vi "Throw Invalid RDMA Configuration Error.vi"(7 "source vi name":string, 8 "error in":errorcluster) -> (0 "error out":errorcluster)   [LabVIEW 2020, in "RDMA.lvlib" / "RDMA Transceiver.lvclass"]
uses:
  RDMA Transceiver.lvclass
  Errors.ctl
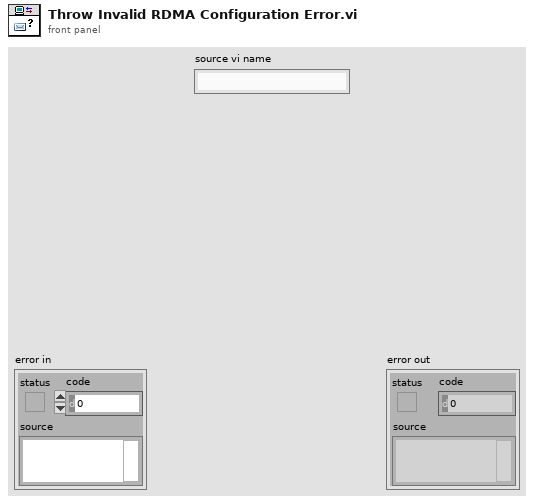
[diagram p1: front panel]
types:
  T1 = typedef "RDMA.lvlib/RDMA Transceiver.lvclass/Errors.ctl" = enum16{"Invalid RDMA Configuration", "Too Many Transfers", "Size Mismatch", "Unknown Setting"}
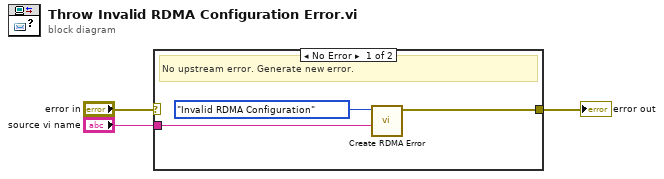
[diagram p0: block diagram]
diagram:
  n1 = case shown="No Error" "error in" {
    selector: "error in" -> [_ w7]
    tunnel: [w5 w7] -> w2
    tunnel: "source vi name" -> [w4 _]
    frame No Error {
      # "No upstream error. Generate new error."
      n2 = call "Create RDMA Error.vi"("source vi name"=w4, "error"=Errors."Invalid RDMA Configuration" ("Error")) -> ("error out"=w5:errorcluster)  [unwired: 8 in, 1 out]
    }
    frame Error {
      # "Upstream error. Pass through."
    }
  }
  "error out" <- w2
